vi "Read Update Period.vi"(11 "ILC in":refnum<class "ILC.lvclass">) -> (2 "Update Period":dbl[unit]=0.1 min=0.001 max=5.0, 3 "ILC out":refnum<class "ILC.lvclass">)   [LabVIEW 2013, in "ILCCommon.lvlib" / "ILC.lvclass"]
uses:
  <userlib>/Common/ILC/ILC/ILC.lvclass
  <userlib>/Common/ILC/ILC/ILC.lvclass/ILC.ctl
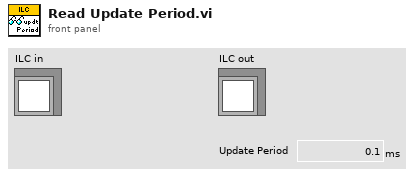
[diagram p1: front panel]
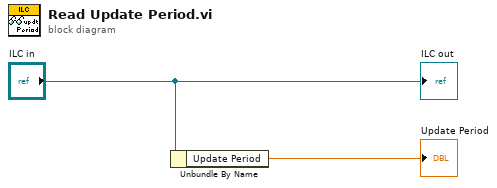
[diagram p0: block diagram]
diagram:
  n1 = Unbundle By Name("ILC in") -> ("Update Period"=→"Update Period":dbl[unit])
  "ILC out" <- "ILC in"
